vi "Acquire Color Image with Skeletal Mapping.vi"() -> ()   [LabVIEW 2011, in "LVH-KinectOne.lvlib"]
doc: "This example demonstrates how to acquire a Body Index frame from the Microsoft Kinect One."
uses:
  vi.lib/LabVIEW Hacker/KinectOne/LVH-KinectOne.lvlib
  vi.lib/LabVIEW Hacker/KinectOne/Private/Initialize Image [Color].vi
  vi.lib/LabVIEW Hacker/KinectOne/Private/kinectRead [ColorFrame].vi
  vi.lib/LabVIEW Hacker/KinectOne/Private/kinectRead [BodyFrame].vi
panel:
  in  "Stop Button":bool
  out "Body Index Image":T1(plugin-control)
  # "LVH Interface for Kinect One \nAcquire Color Image With Skeletal Mapping Example\n\nThis example demonstrates how to acquire a color image data from the Kinect and overlay skeletal \ndata on the image.\n\n1. Make sure you have the Kinect SDK 2.0 installed.\n2. Connect the Kinect sensor to the computer via USB.\n3. Click the Run button.\n4. Stand in front of the Kinect sensor.\n\nHave feedback or need help?  Visit the LabVIEW Hacker forums at www.labviewhacker.com/forums/kinect"
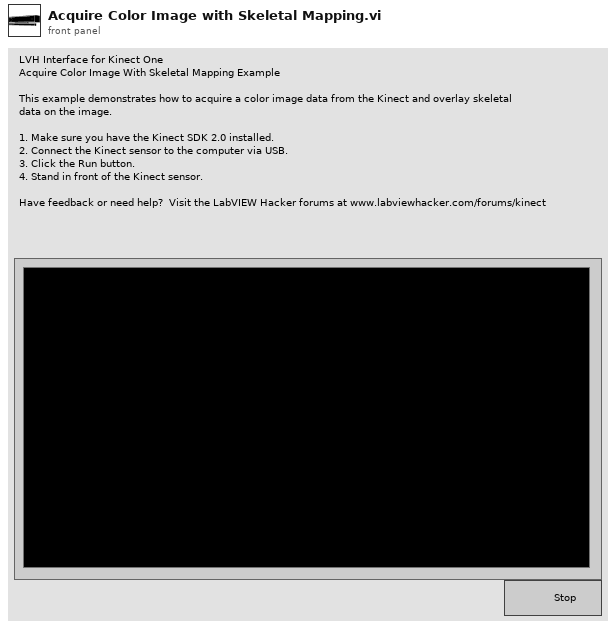
[diagram p1: front panel]
types:
  T1 = typedef "IMAQ Image.ctl" = refnum<image>
  T2 = typedef "LVH-KinectOne.lvlib/KinectSensor References.ctl" = cluster{"KinectSensor":refnum<k24>, "MultiSourceFrameReader":refnum<k24>, "BodyFrameDataInterface":refnum<k24>}
  T3 = typedef "LVH-KinectOne.lvlib/BodyData.ctl" = cluster{"ClippedEdges":T4, "HandLeftConfidence":T5, "HandLeftState":T6, "HandRightConfidence":T7, "HandRightState":T8, "IsRestricted":bool, "IsTracked":bool, "JointOrientations":refnum<k24>, "Joints":refnum<k24>, "Lean":refnum<k24>, "LeanTrackingState":T9, "TrackingId":u64}
  T4 = typedef "LVH-KinectOne.lvlib/ClippedEdges.ctl" = enum16{"None", "Right", "Left", "Top", "Bottom"}
  T5 = typedef "LVH-KinectOne.lvlib/HandLeftConfidence.ctl" = enum16{"Low", "High"}
  T6 = typedef "LVH-KinectOne.lvlib/HandLeftState.ctl" = enum16{"Unknown", "NotTracked", "Open", "Closed", "Lasso"}
  T7 = typedef "LVH-KinectOne.lvlib/HandRightConfidence.ctl" = enum16{"Low", "High"}
  T8 = typedef "LVH-KinectOne.lvlib/HandRightState.ctl" = enum16{"Unknown", "NotTracked", "Open", "Closed", "Lasso"}
  T9 = typedef "LVH-KinectOne.lvlib/LeanTrackingState.ctl" = enum16{"NotTracked", "Inferred", "Tracked"}
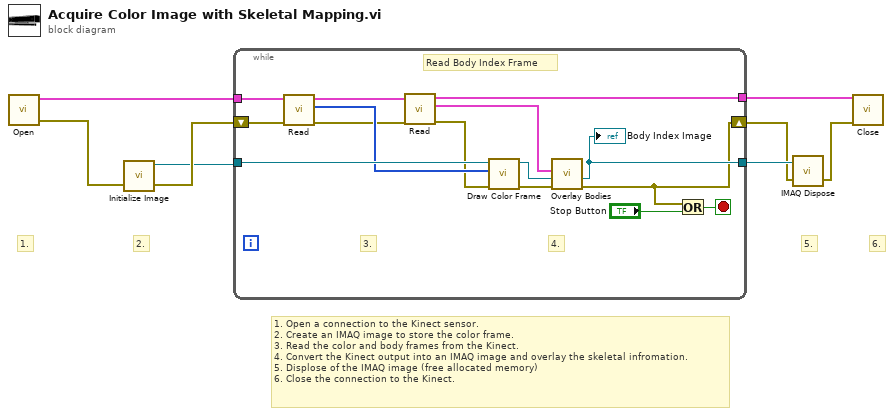
[diagram p0: block diagram]
diagram:
  # "1. Open a connection to the Kinect sensor.\n2. Create an IMAQ image to store the color frame.\n3. Read the color and body frames from the Kinect.\n4. Convert the Kinect output into an IMAQ image and overlay the skeletal infromation.\n5. Displose of the IMAQ image (free allocated memory)\n6. Close the connection to the Kinect."
  # "6."
  # "5."
  # "2."
  # "1."
  n1 = call "Open.vi"() -> ("Error Out"=w4:errorcluster, "KinectSensor References out"=w5:T2)  [unwired: 10 in]
  n2 = call-poly "Initialize Image.vi"("Error In"=w4) -> ("Error Out"=w3:errorcluster, "Color Image"=w2:T1)  [unwired: 9 in]
  n3 = while {
    tunnel: w5 -> [w23]
    shift-right: [w20] -> w7
    shift-left: w3 -> [w22]
    tunnel: w2 -> [w14]
    tunnel: [w21] -> w8
    tunnel: [w16] -> w1
    stop <- w19 stop-if-true
    # "4."
    # "3."
    # "Read Body Index Frame"
    n4 = call-poly "Read.vi"("Error In"=w22, "KinectSensor References in"=w23) -> ("Error Out"=w10:errorcluster, "frameData"=w11:u32[], "KinectSensor References out"=w17:T2)  [unwired: 7 in]
    n5 = call-poly "Read.vi"("error in (no error)"=w10, "KinectSensor References in"=w17) -> ("error out"=w9:errorcluster, "Body Data"=w12:T3[], "KinectSensor References out"=w16:T2)  [unwired: 7 in]
    n6 = call "Draw Color Frame.vi"("Error In"=w9, "U32 Array"=w11, "Image"=w14) -> ("Error Out"=w15:errorcluster, "Image Out"=w13:T1)  [unwired: 7 in]
    n7 = call "Overlay Bodies.vi"("Error In"=w15, "Image"=w13, "Body Data"=w12) -> ("Error Out"=w20:errorcluster, "Image Out"=w21:T1)  [unwired: 7 in]
    "Body Index Image" <- w21
    n8 = Or(x=w20, y="Stop Button") -> (x .or. y?=w19:bool)
  }
  n9 = call "IMAQ Dispose"("Image"=w8, "error in (no error)"=w7) -> ("error out"=w6:errorcluster)  [unwired: 4 in]
  n10 = call "Close.vi"("Error In"=w6, "KinectSensor References"=w1) -> ()  [unwired: 9 in, 1 out]
